vi "Indexer.vi"(10 "Fire":bool=TRUE, 11 "Shooter States":T1) -> (3 "Indexer Value":dbl)   [LabVIEW 2015]
uses:
  Typedefs/Shooter States.ctl
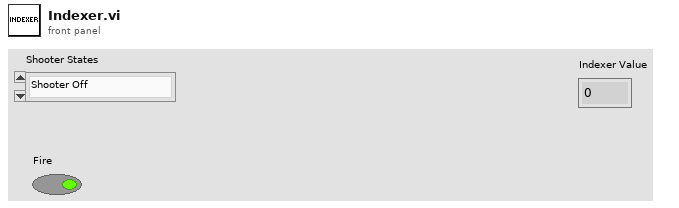
[diagram p1: front panel]
types:
  T1 = typedef "Shooter States.ctl" = enum16{"Shooter Off", "Shooter Far", "Shooter Close", "Shooter Intermediate"}
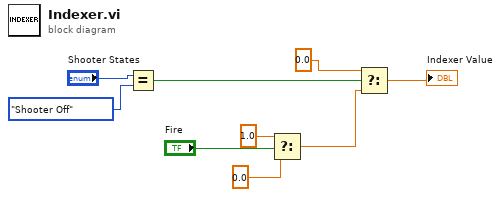
[diagram p0: block diagram]
diagram:
  n1 = Equal?(x="Shooter States", y=Shooter_States."Shooter Off" ("Shooter States 2")) -> (x = y?=w6:bool)
  n2 = Select(t=1.0, s="Fire", f=0.0) -> (s? t:f=w2:dbl)
  n3 = Select(t=0.0, s=w6, f=w2) -> (s? t:f=→"Indexer Value":dbl)
